vi "Waveform.Task.GetRate.vi"(8 "error in (no error)":errorcluster, 11 "Waveform Section Ref in":T1 format="%.0x") -> (0 "error out":errorcluster, 2 "Task Rate":dbl, 3 "Waveform Section Ref out":T1 format="%.0x")   [LabVIEW 2015, in "Waveform-Processing-Custom-Device System Explorer.lvlib"]
uses:
  Waveform-Processing-Custom-Device System Explorer.lvlib
  <vilib>/NI Veristand/Custom Device API/Custom Device Item Ref.ctl
  NationalInstruments.VeriStand.SystemStorage
  Shared/Constants.vi
  <vilib>/NI Veristand/Custom Device API/Get Item Property (Dependent Node Pointer).vi
  <vilib>/NI VeriStand/Custom Device API/Custom Device API.lvlib
  Shared/Waveform-Processing-Custom-Device Shared.lvlib
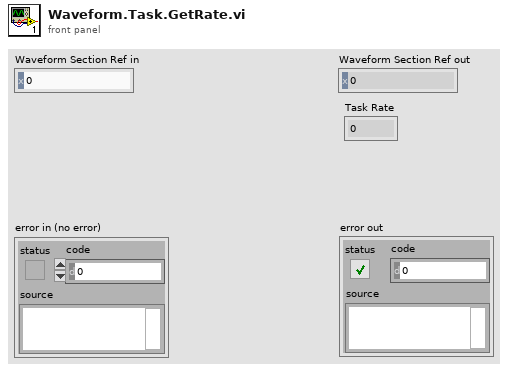
[diagram p1: front panel]
types:
  T1 = typedef "Custom Device API.lvlib/Custom Device Item Ref.ctl" = u64
  T2 = typedef "Custom Device API.lvlib/Custom Device Pointer.ctl" = refnum<k24>
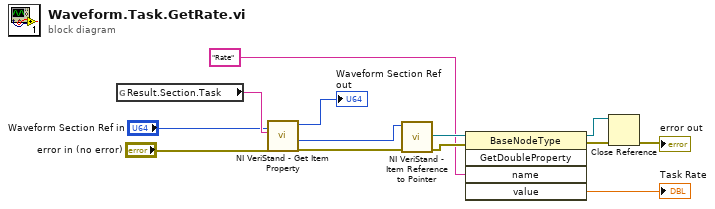
[diagram p0: block diagram]
diagram:
  n1 = global read "Constants.vi" "Result.Section.Task"() -> (w8:string)
  n2 = call-poly <vilib>:"NI VeriStand - Get Item Property.vi"("error in (no error)"="error in (no error)", "Property Name"=w8, "Item Ref in"="Waveform Section Ref in") -> ("error out"=w9:errorcluster, "Dependent Node Ref"=w10:T1, "Item Ref out"=→"Waveform Section Ref out":T1)  [unwired: 5 in, 1 out]
  n3 = call <vilib>:"NI VeriStand - Item Reference to Pointer.vi"("error in (no error)"=w9, "Item Ref in"=w10) -> ("error out"=w12:errorcluster, "Node Pointer"=w11:T2)  [unwired: 6 in, 2 out]
  n4 = invoke class="BaseNodeType" method="GetDoubleProperty"(reference=w11, error in=w12, "name"="Rate") -> (reference out=w3:T2, error out=w4:errorcluster, "value"=→"Task Rate":dbl)  [unwired: 2 in, 2 out]
  n5 = Close Reference(reference=w3, error in (no error)=w4) -> (error out=→"error out":errorcluster)
